vi "Error Log internals.vi"(8 "error in (no error)":errorcluster, 10 "Log in":refnum<class "Log.lvclass">, 11 "Object in":refnum<class>) -> (0 "error out":errorcluster, 2 "Log out":refnum<class "Log.lvclass">)   [LabVIEW 2026, in "TALOS.lvlib"]
uses:
  TALOS.lvlib
  Classes/Log/Log.lvclass
  Ancestor/Ancestor/Ancestor.lvclass
  Ancestor/Ancestor/Ancestor.lvclass/Ancestor.ctl
  Classes/Log/Log.lvclass/Log.ctl
  Ancestor/Ancestor/Read ID.vi
  <vilib>/AdvancedString/Delimited String to 1D String Array.vi
  <vilib>/AdvancedString/Delimited String to 1D String Array (string).vi
  Classes/Log/Write.vi
  Generate Error.vi
  Date n Time.vi
  FGV/Error Memory/Get Error Description.vi
  Get PC name.vi
  <vilib>/Utility/error.llb/Clear Errors.vi
  FGV/Error Memory/Error Memory Core.vi
  Circus Root Path.vi
  FGV/Error Memory/Error Crt Lvl checker.vi
  FGV/Error Memory/Error Memory Core.vi/40c8088d-b597-4017-91af-faa98e00292e.vi
  FGV/Error Memory/Error Memory Core.vi/d4a3ab98-063c-4e44-b43d-fbdcfe6c2be2.vi
  <vilib>/Utility/LVClass/Get LV Class Name.vi
  Classes/Log/Rotate.vi
  Global Memory.vi
  Is in Packed Library.vi
  TALOS Root path.vi
  Read CSV worksheet.vi
  Global Constants.vi
  <vilib>/Utility/error.llb/General Error Handler.vi
  <vilib>/Comparison/Equal/Equal Functor/Equal Functor.lvclass
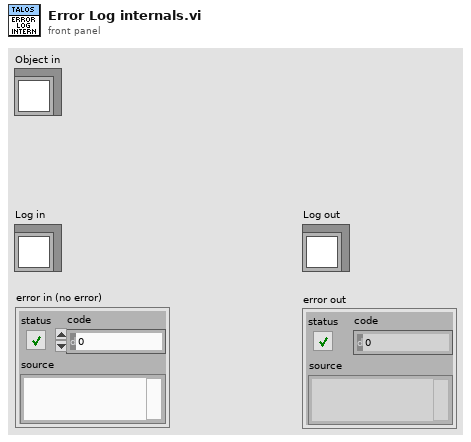
[diagram p1: front panel]
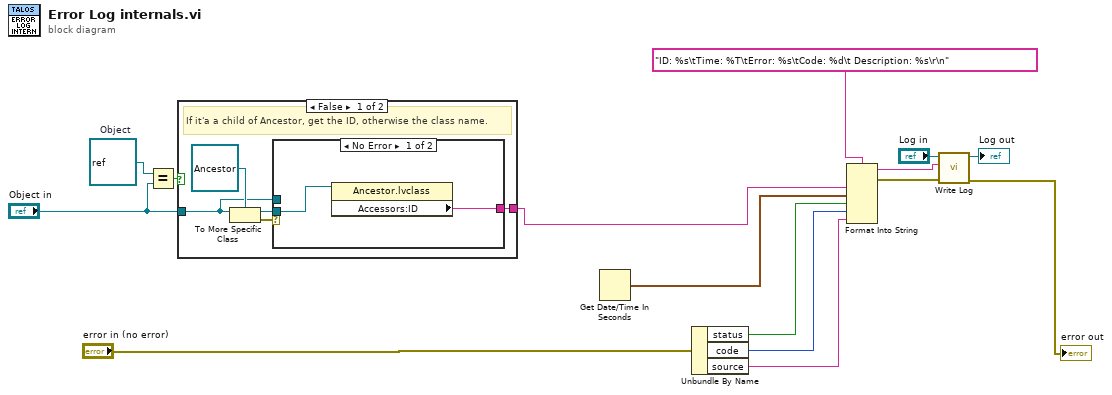
[diagram p0: block diagram]
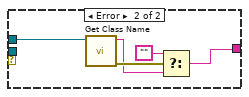
[diagram p2: hidden frame]
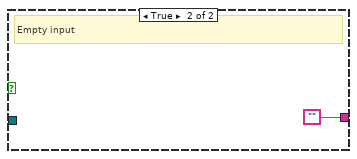
[diagram p3: hidden frame]
diagram:
  w14 = refnum<class> refnum  # Object
  n1 = Equal?(x=w14, y="Object in") -> (x = y?=w13:bool)
  n2 = case shown="False" w13 {
    tunnel: [w20 ""] -> w9
    tunnel: "Object in" -> [w16 _]
    frame False {
      # "If it'a a child of Ancestor, get the ID, otherwise the class name."
      n3 = To More Specific Class(target class=refnum<class "Ancestor.lvclass"> refnum ("TALOS.lvlib:Ancestor.lvlib:Ancestor.lvclass"), reference=w16) -> (specific class reference=w18:refnum<class "Ancestor.lvclass">, error out=w17:errorcluster)  [unwired: 1 in]
      n4 = case shown="No Error" w17 {
        tunnel: [w22 w24] -> w20
        tunnel: w18 -> [w21 _]
        tunnel: w16 -> [_ w27]
        frame No Error {
          n5 = property class="Ancestor.lvclass"(reference=w21) -> ("Accessors:ID"=w22:string)  [unwired: 1 in, 2 out]
        }
        frame Error {
          n6 = call "Get Class Name.vi"("object"=w27) -> ("error out"=w26:errorcluster, "Class Name"=w25:string)  [unwired: 9 in]
          n7 = Select(t="", s=w26, f=w25) -> (s? t:f=w24:string)
        }
      }
    }
    frame True {
      # "Empty input"
    }
  }
  n8 = Get Date/Time In Seconds() -> (seconds since 1Jan1904=w8:timestamp)
  n9 = Unbundle By Name("error in (no error)") -> ("status"=w7:bool, "code"=w6:i32, "source"=w5:string)
  n10 = Format Into String(format string="ID: %s\tTime: %T\tError: %s\tCode: %d\t Description: %s\r\n", w9, w8, w7, w6, w5) -> (resulting string=w3:string, error out=w2:errorcluster)  [unwired: 2 in]
  n11 = call "Write Log.vi"("error in (no error)"=w2, "Text"=w3, "Log in"="Log in") -> ("error out"=→"error out":errorcluster, "Log out"=→"Log out":refnum<class "Log.lvclass">)  [unwired: 7 in]
